vi "Balance_Sweep_Post_Proc.vi"() -> ()   [LabVIEW 2022 SP3]
uses:
  Controls/Live Balance Data.ctl
  <vilib>/Analysis/1siggen.llb/Ramp Pattern by Samples.vi
  <vilib>/Analysis/NI_AALBase.lvlib
  <vilib>/Analysis/1siggen.llb/Ramp Pattern by Delta.vi
  <vilib>/gmath/NI_Gmath.lvlib
  <vilib>/Analysis/NI_AALPro.lvlib
  <vilib>/Analysis/2dsp.llb/1D Cross Correlation (DBL).vi
  <vilib>/Analysis/NI_AAL_SigProc.lvlib
panel:
  out "XY Graph 5":T1(graph)
  out "XY Graph 4":T1(graph)
  out "XY Graph":cluster{dbl[], dbl[]}[](graph)
  out "Array":dbl[](array[numeric])
  out "XY Graph 2":cluster{dbl[], dbl[]}[](graph)
  out "Array 2":i32[](array[numeric])
  in  "Live Balance Data Array":path[](array[path])
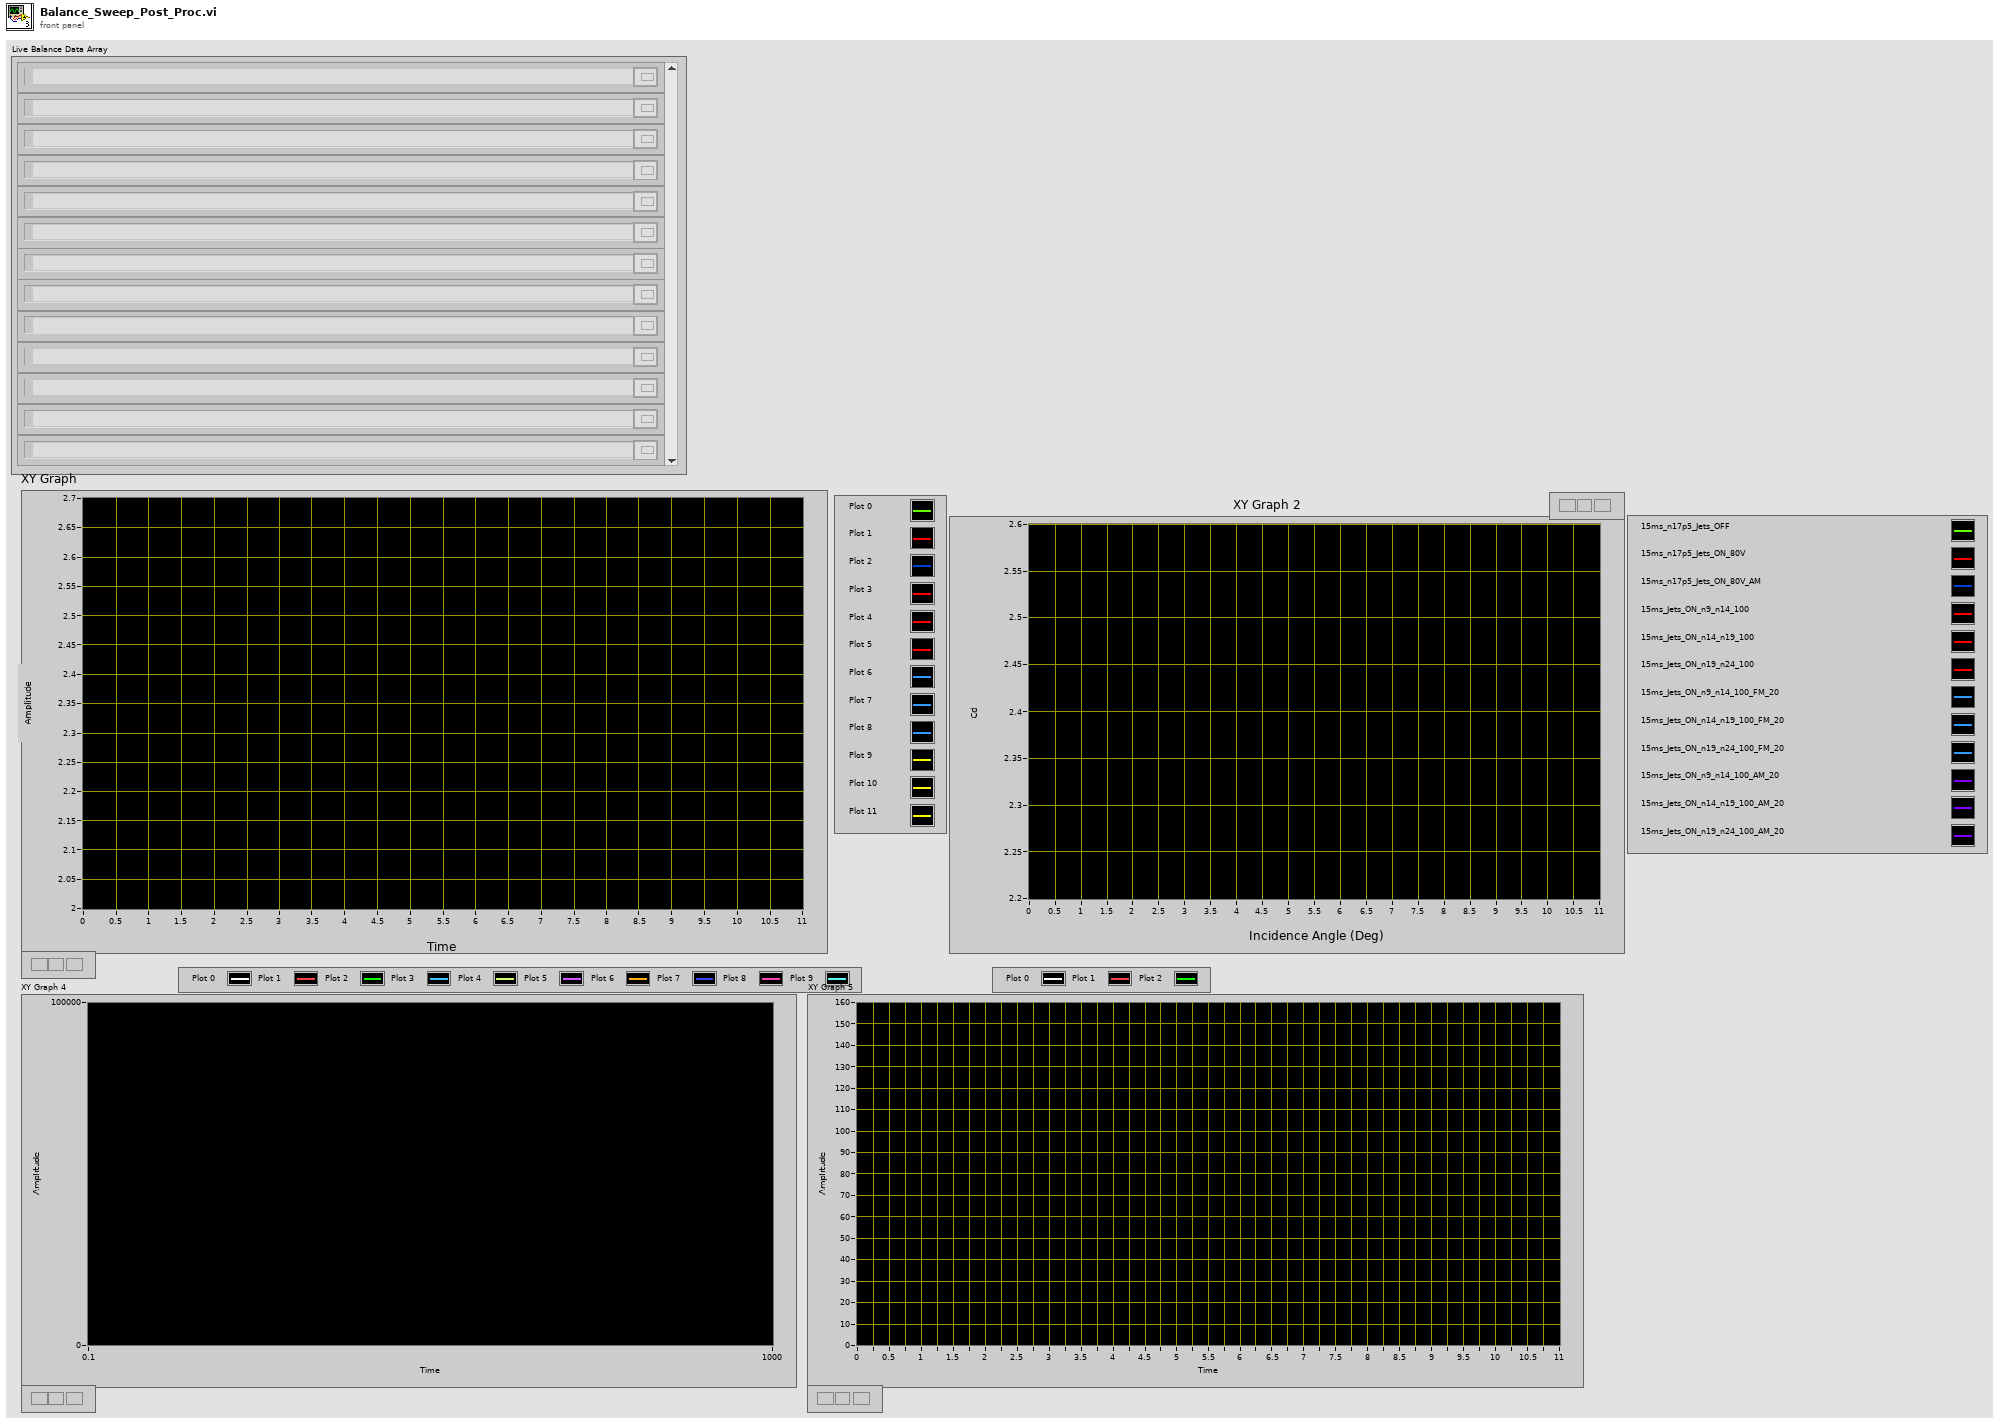
[diagram p1: front panel]
types:
  T1 = cluster{"Ramp Pattern":dbl[], "Power Spectrum (V^2 rms)":dbl[]}[]
  T2 = enum16{"big-endian, network order", "native, host order", "little-endian"}
  T3 = typedef "Live Balance Data.ctl" = cluster{"AS Freq (Hz)":dbl, "Time (s)":dbl[], "Pressure 2 (V)":dbl[], "Pressure 3 (V)":dbl[], "Wind Speed (m/s)":dbl[], "Balance AS Freq (Hz)":dbl[], "Live Angle (deg)":dbl[], "Live Angle An(deg)":dbl[], "Balance Loads":cluster{"Lift (%)":dbl[], "Lift (N)":dbl[], "Pitch (%)":dbl[], "Pitch (Nm)":dbl[], "Drag (%)":dbl[], "Drag (N)":dbl[], "Side (%)":dbl[], "Side (N)":dbl[], "Yaw (%)":dbl[], "Yaw (Nm)":dbl[], "Roll (%)":dbl[], "Roll (Nm)":dbl[]}, "Pressure 1 (V)":dbl[], "Pressure SJ (V)":dbl[]}
  T4 = cluster{"Ramp Pattern":dbl[], "Power Spectrum (V^2 rms)":dbl[]}
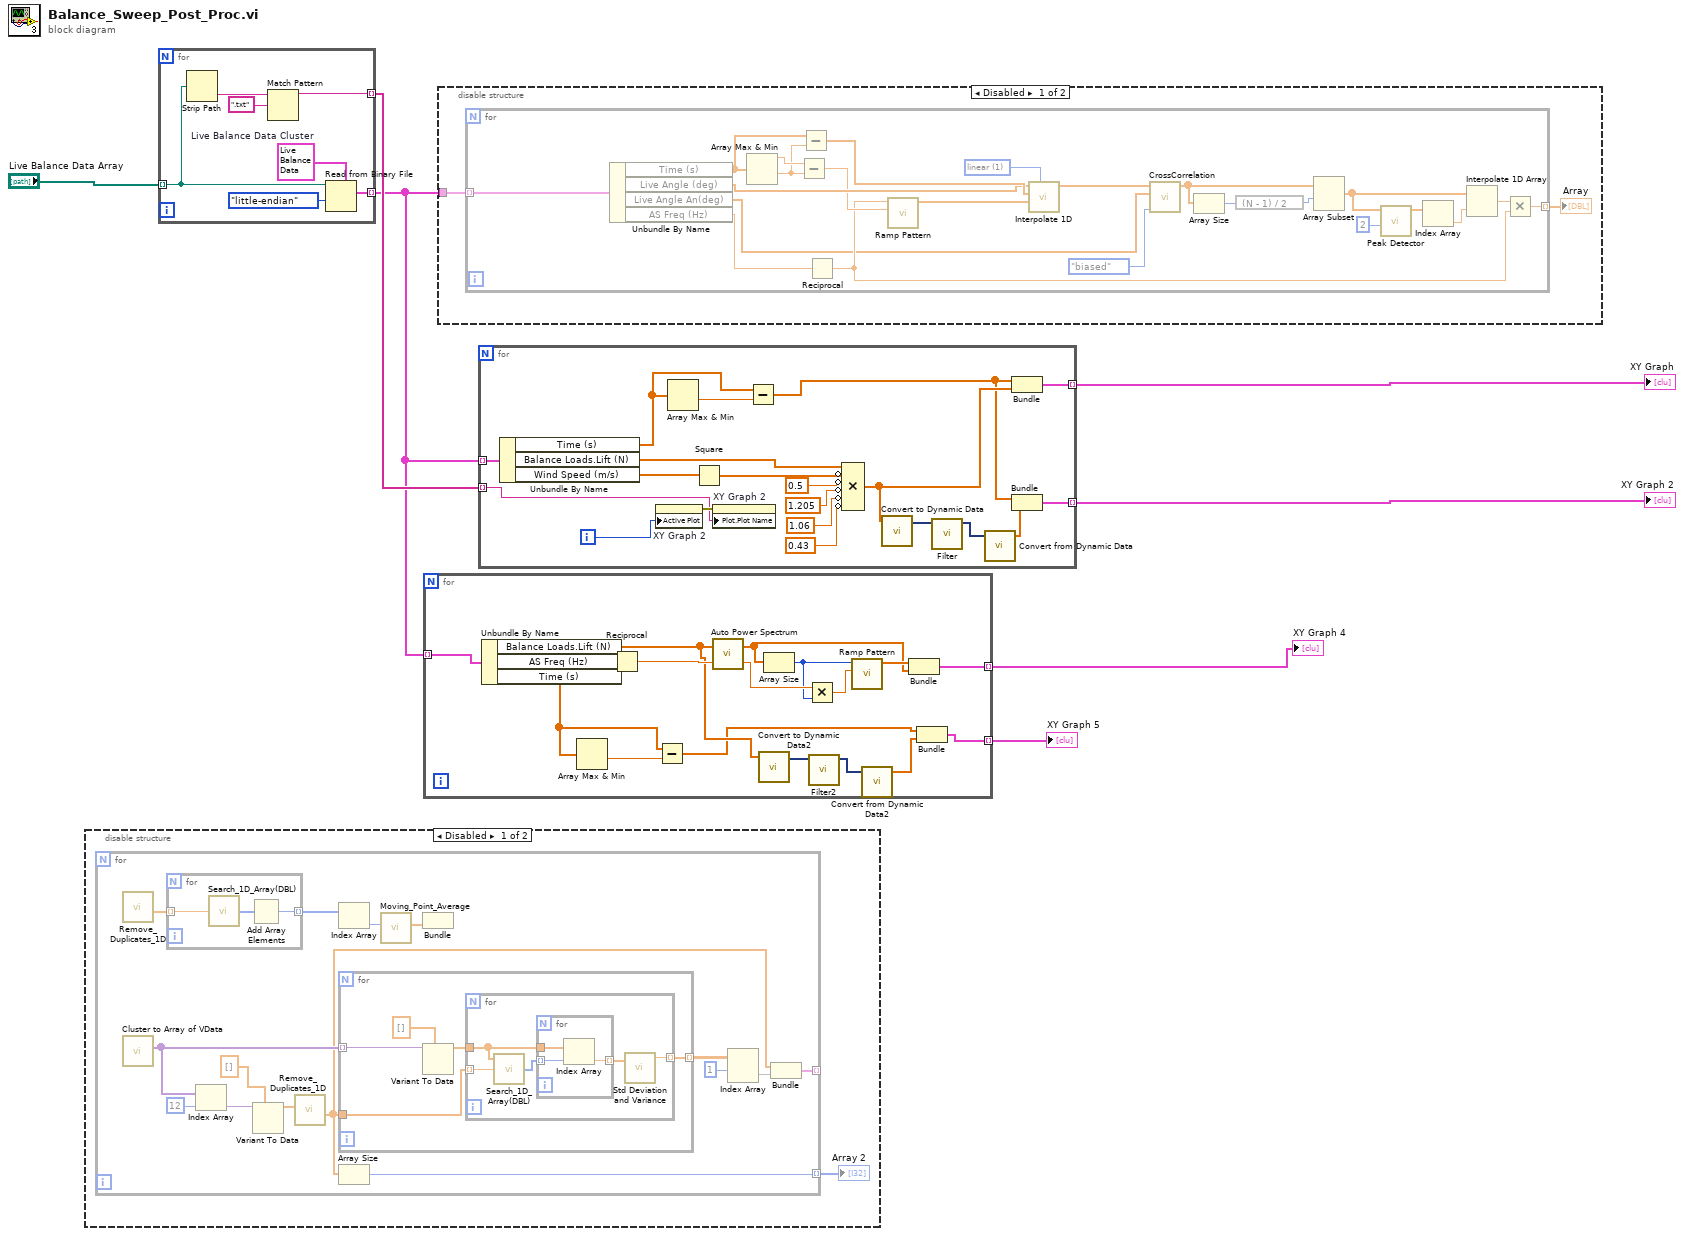
[diagram p0: block diagram]
diagram:
  n1 = disable-structure shown="Disabled" {
    frame Disabled {
      n2 = for {
        tunnel: [w21] -> w9 mode=indexing
        tunnel: [w14] -> w8 mode=indexing
        n3 = call "Remove_Duplicates_1D.vi"() -> ("Unique Array"=w10:dbl[])  [unwired: 10 in, 1 out]
        n4 = call "Cluster to Array of VData.vi"() -> ("Array of VData"=w19:variant[])  [unwired: 10 in, 1 out]
        n5 = for {
          tunnel: w10 -> [w27] mode=indexing
          tunnel: [w25] -> w11 mode=indexing
          n6 = call "Search_1D_Array(DBL).vi"("Element Data"=w27) -> ("Indicies of Elements"=w26:i32[])  [unwired: 7 in, 1 out]
          n7 = Add Array Elements(numeric array=w26) -> (sum=w25:i32)
        }
        n8 = Index Array(array=w19, index=12) -> (element=w23:variant)
        n9 = Variant To Data(type=dbl[] [] ("subarray"), Variant=w23) -> (data=w20:dbl[])  [unwired: 1 in, 1 out]
        n10 = call "Remove_Duplicates_1D.vi"("Input Array"=w20) -> ("Unique Array"=w15:dbl[])  [unwired: 9 in, 1 out]
        n11 = Index Array(array=w11) -> (element=w13:i32)  [unwired: 1 in]
        n12 = for {
          tunnel: w15 -> [w32]
          tunnel: [w31] -> w18 mode=indexing
          tunnel: w19 -> [w30] mode=indexing
          n13 = Variant To Data(type=dbl[] [] ("subarray"), Variant=w30) -> (data=w28:dbl[])  [unwired: 1 in, 1 out]
          n14 = for {
            tunnel: w28 -> [w36]
            tunnel: w32 -> [w37] mode=indexing
            tunnel: [w34] -> w31 mode=indexing
            n15 = call "Search_1D_Array(DBL).vi"("Array"=w36, "Element Data"=w37) -> ("Indicies of Elements"=w33:i32[])  [unwired: 6 in, 1 out]
            n16 = for {
              tunnel: w36 -> [w40]
              tunnel: w33 -> [w39] mode=indexing
              tunnel: [w38] -> w35 mode=indexing
              n17 = Index Array(array=w40, index=w39) -> (element=w38:dbl)
            }
            n18 = call <vilib>:"Std Deviation and Variance.vi"("X"=w35) -> ("mean"=w34:dbl)  [unwired: 1 in, 2 out]
          }
        }
        n19 = Array Size(array=w15) -> (size(s)=w21:i32)
        n20 = call "Moving_Point_Average.vi"("Averaging Points"=w13) -> ("Moving Average of X"=w12:dbl[])  [unwired: 10 in]
        n21 = Bundle("Moving Average of X"=w12) -> ()  [unwired: 2 in, 1 out]
        n22 = Index Array(array=w18, index (row)=1) -> (element=w16:dbl[])  [unwired: 1 in]
        n23 = Bundle("Unique Array"=w15, w16) -> (w14:cluster{"Unique Array":dbl[], dbl[]})  [unwired: 1 in]
      }
      "Array 2" <- w9
    }
    frame Enabled {
    }
  }
  n24 = for {
    tunnel: "Live Balance Data Array" -> [w46] mode=indexing
    tunnel: [w43] -> w4 mode=indexing
    tunnel: [w41] -> w3 mode=indexing
    w42 = T3 {"AS Freq (Hz)"=0.0, "Time (s)"=[], "Pressure 2 (V)"=[], "Pressure 3 (V)"=[], "Wind Speed (m/s)"=[], "Balance AS Freq (Hz)"=[], "Live Angle (deg)"=[], "Live Angle An(deg)"=[], "Balance Loads"={"Lift (%)"=[], "Lift (N)"=[], "Pitch (%)"=[], "Pitch (Nm)"=[], "Drag (%)"=[], "Drag (N)"=[], "Side (%)"=[], "Side (N)"=[], "Yaw (%)"=[], "Yaw (Nm)"=[], "Roll (%)"=[], "Roll (Nm)"=[]}, "Pressure 1 (V)"=[], "Pressure SJ (V)"=[]}  # Live Balance Data Cluster
    n25 = Strip Path(path=w46) -> (name=w45:string)  [unwired: 1 out]
    n26 = Match Pattern(string=w45, regular expression=".txt") -> (before substring=w43:string)  [unwired: 1 in, 3 out]
    n27 = Read from Binary File(5:w42, 9:T2."little-endian" ("byte order (0:big-endian, network order)"), 11:w46) -> (2:w41:T3)  [unwired: 3 in, 3 out]
  }
  n28 = for {
    tunnel: w3 -> [w63] mode=indexing
    tunnel: [w57] -> w2 mode=indexing
    tunnel: [w55] -> w1 mode=indexing
    n29 = Unbundle By Name(w63) -> ("Balance Loads.Lift (N)"=w49:dbl[], "AS Freq (Hz)"=w64:dbl, "Time (s)"=w50:dbl[])
    n30 = Array Max & Min(array=w50) -> (min value=w51:dbl)  [unwired: 3 out]
    n31 = Reciprocal(x=w64) -> (1/x=w56:dbl)
    n32 = Subtract(x=w50, y=w51) -> (x-y=w48:dbl[])
    n33 = call <vilib>:"Auto Power Spectrum.vi"("dt"=w56, "Signal (V)"=w49) -> ("df"=w62:dbl, "Power Spectrum (V^2 rms)"=w58:dbl[])
    n34 = call "Convert to Dynamic Data2"("Array"=w49) -> ("Dynamic Data Type"=w53:dynamicdata)  [unwired: 3 in]
    n35 = Array Size(array=w58) -> (size(s)=w61:i32)
    n36 = Multiply(x=w62, y=w61) -> (x*y=w60:dbl)
    n37 = call "Filter2"("Signal"=w53) -> ("Filtered Signal"=w54:dynamicdata)  [unwired: 9 in, 1 out]
    n38 = call-poly <vilib>:"Ramp Pattern.vi"("end"=w60, "samples"=w61) -> ("Ramp Pattern"=w59:dbl[])  [unwired: 8 in, 1 out]
    n39 = call "Convert from Dynamic Data2"("Dynamic Data Type"=w54) -> ("Array"=w52:dbl[])  [unwired: 3 in]
    n40 = Bundle("Ramp Pattern"=w59, "Power Spectrum (V^2 rms)"=w58) -> (w57:T4)  [unwired: 1 in]
    n41 = Bundle(w48, "Array"=w52) -> (w55:cluster{dbl[], "Array":dbl[]})  [unwired: 1 in]
  }
  "XY Graph 4" <- w2
  "XY Graph 5" <- w1
  n42 = disable-structure shown="Disabled" {
    disable-tunnel: w3 -> [w66 _]
    frame Disabled {
      n43 = for {
        tunnel: w66 -> [w89] mode=indexing
        tunnel: [w67] -> w65 mode=indexing
        w83 = 1 items=["nearest", "linear", "spline", "cubic Hermite", "Lagrange"] ("method")
        n44 = Unbundle By Name(w89) -> ("Time (s)"=w87:dbl[], "Live Angle (deg)"=w82:dbl[], "Live Angle An(deg)"=w68:dbl[], "AS Freq (Hz)"=w85:dbl)
        n45 = Array Max & Min(array=w87) -> (max value=w88:dbl, min value=w86:dbl)  [unwired: 2 out]
        n46 = Subtract(x=w88, y=w86) -> (x-y=w81:dbl)
        n47 = Subtract(x=w87, y=w86) -> (x-y=w84:dbl[])
        n48 = Reciprocal(x=w85) -> (1/x=w70:dbl)
        n49 = call-poly <vilib>:"Ramp Pattern.vi"("end"=w81, "delta"=w70) -> ("Ramp Pattern"=w69:dbl[])  [unwired: 7 in, 2 out]
        n50 = call <vilib>:"Interpolate 1D.vi"("method"=w83, "xi"=w69, "X"=w84, "Y"=w82) -> ("yi"=w79:dbl[])  [unwired: 5 in, 2 out]
        n51 = call-poly <vilib>:"CrossCorrelation.vi"("normalization"=enum32{"none", "unbiased", "biased"}."biased", "Y"=w68, "X"=w79) -> ("Rxy"=w76:dbl[])  [unwired: 7 in, 1 out]
        n52 = Array Size(array=w76) -> (size(s)=w78:i32)
        n53 = expression code="(N - 1) / 2"(w78) -> (w77:i32)
        n54 = Array Subset(array=w76, index=w77) -> (w73:dbl[])  [unwired: 1 in]
        n55 = call <vilib>:"Peak Detector.vi"("width"=2, "X"=w73) -> ("Locations"=w74:dbl[])  [unwired: 5 in, 4 out]
        n56 = Index Array(array=w74) -> (element=w72:dbl)  [unwired: 1 in]
        n57 = Interpolate 1D Array(1:w72, 2:w73) -> (0:w71:dbl)
        n58 = Multiply(x=w71, y=w70) -> (x*y=w67:dbl)
      }
      "Array" <- w65
    }
    frame Enabled {
    }
  }
  n59 = for {
    tunnel: w3 -> [w109] mode=indexing
    tunnel: [w108] -> w5 mode=indexing
    tunnel: [w107] -> w6 mode=indexing
    tunnel: w4 -> [w93] mode=indexing
    i -> [w95]
    n60 = Unbundle By Name(w109) -> ("Time (s)"=w92:dbl[], "Balance Loads.Lift (N)"=w100:dbl[], "Wind Speed (m/s)"=w106:dbl[])
    n61 = property on="XY Graph 2" class="XYGraph (strict)"("Active Plot"=w95) -> (error out=w94:errorcluster)  [unwired: 2 in, 1 out]
    n62 = Array Max & Min(array=w92) -> (min value=w91:dbl)  [unwired: 3 out]
    n63 = Square(x=w106) -> (x^2=w105:dbl[])
    n64 = property on="XY Graph 2" class="XYGraph (strict)"(error in=w94, "Plot.Plot Name"=w93) -> ()  [unwired: 1 in, 2 out]
    n65 = Subtract(x=w92, y=w91) -> (x-y=w90:dbl[])
    n66 = Compound Arithmetic op=MULTIPLY(w100, invert w105, invert 0.5 ("Numeric"), invert 1.205 ("value"), invert 1.06 ("value"), invert 0.43 ("value")) -> (w97:dbl[])
    n67 = call "Convert to Dynamic Data"("Array"=w97) -> ("Dynamic Data Type"=w99:dynamicdata)  [unwired: 3 in]
    n68 = call "Filter"("Signal"=w99) -> ("Filtered Signal"=w98:dynamicdata)  [unwired: 9 in, 1 out]
    n69 = call "Convert from Dynamic Data"("Dynamic Data Type"=w98) -> ("Array"=w96:dbl[])  [unwired: 3 in]
    n70 = Bundle(w90, w97) -> (w107:cluster{dbl[], dbl[]})  [unwired: 1 in]
    n71 = Bundle(w90, "Array"=w96) -> (w108:cluster{dbl[], "Array":dbl[]})  [unwired: 1 in]
  }
  "XY Graph" <- w6
  "XY Graph 2" <- w5
